vi "4-5 reverse.vi"() -> ()   [LabVIEW 2014]
doc: "This VI illustrates how to acquire a finite number of samples from a specified device. It requires the use of a microphone attached to the sound card. You can specify the number of samples to acquire, sample rate, number of channels and a bit rate per sample.\n------------------------------------\nAuther: Koji Ohashi\nCopyright (c) 2020 Japan LabVIEW Users Group, Volunteer members.\nThis VI is released under the MIT License.\nhttp://opensource.org/licenses/mit-license.php\n------------------------------------"
uses:
  <vilib>/sound2/lvsound2.llb/Sampling Mode.ctl
  <vilib>/sound2/lvsound2.llb/Sound Input Read (DBL).vi
  <vilib>/sound2/lvsound2.llb/Sound Output Write (DBL).vi
  <vilib>/sound2/lvsound2.llb/Sound Data Format.ctl
panel:
  out "Sound Output":waveform(dbl)[](graph)
  in  "Recording Time (sec)":dbl=5.0
  in  "Sound Format":T1={"sample rate (S/s)"=22050.0, "number of channels"=2, "bits per sample"=16}
  in  "device ID (Out)":u32
  in  "Device ID":u32
  out "Sound Input":waveform(dbl)[](graph)
  out "Number of Samples/ch":i32=10000
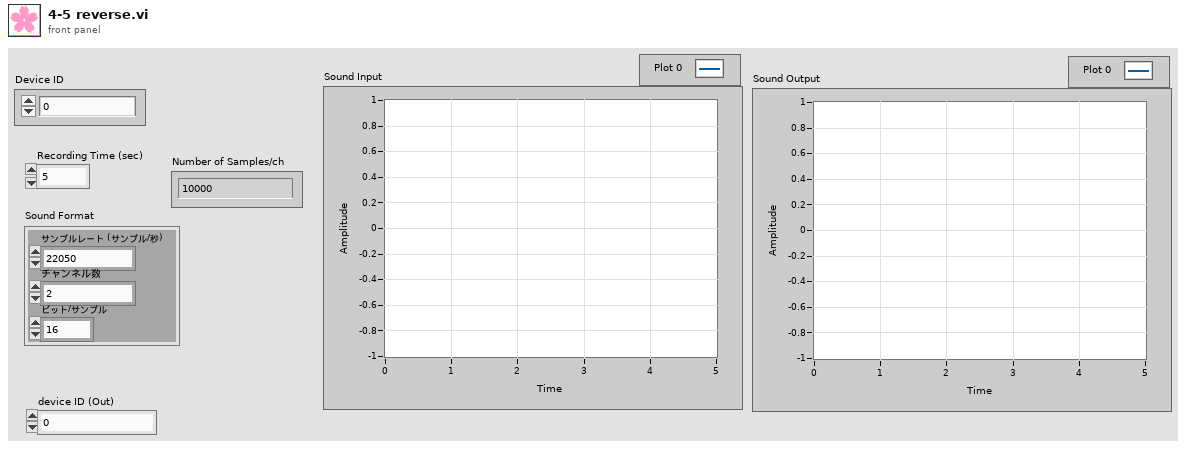
[diagram p1: front panel]
types:
  T1 = typedef "Sound Data Format.ctl" = cluster{"sample rate (S/s)":dbl, "number of channels":i32, "bits per sample":i32}
  T2 = typedef "Sampling Mode.ctl" = i32
  T3 = typedef "Sound Input Task ID.ctl" = u32
  T4 = typedef "Sound Output Task ID.ctl" = u32
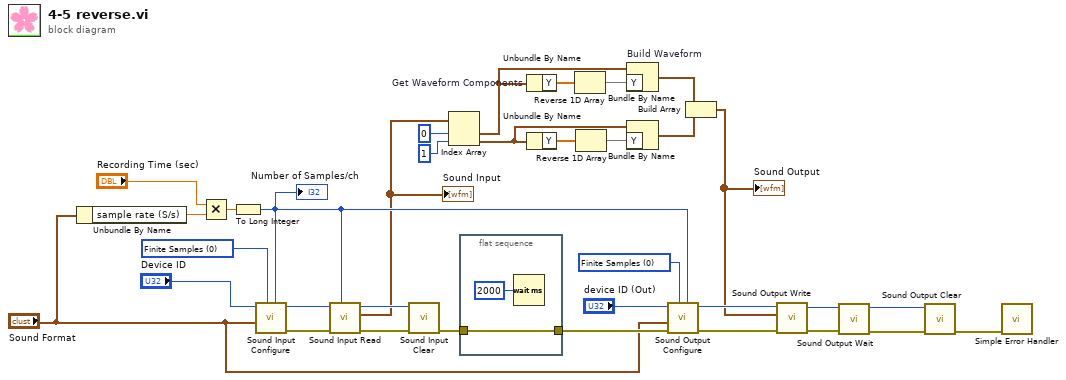
[diagram p0: block diagram]
diagram:
  w23 = T2 0 items=["Finite Samples", "Continuous Samples"] ("sample mode")
  w31 = T2 0 items=["Finite Samples", "Continuous Samples"] ("sample mode")
  n1 = Unbundle By Name("Sound Format") -> ("sample rate (S/s)"=w15:dbl)
  n2 = Multiply(x="Recording Time (sec)", y=w15) -> (x*y=w14:dbl)
  n3 = To Long Integer(number=w14) -> (32bit integer=w13:i32)
  "Number of Samples/ch" <- w13
  n4 = call <vilib>:"Sound Input Configure.vi"("number of samples/ch"=w13, "sample mode"=w31, "sound format"="Sound Format", "device ID"="Device ID") -> ("error out"=w34:errorcluster, "task ID"=w32:T3)  [unwired: 6 in]
  n5 = call-poly <vilib>:"Sound Input Read.vi"("number of samples/ch"=w13, "error in (no error)"=w34, "task ID"=w32) -> ("error out"=w29:errorcluster, "data"=w2:waveform(dbl)[], "task ID out"=w30:T3)  [unwired: 6 in]
  "Sound Input" <- w2
  n6 = call <vilib>:"Sound Input Clear.vi"("error in (no error)"=w29, "task ID"=w30) -> ("error out"=w28:errorcluster)  [unwired: 9 in]
  n7 = Index Array "Index Array"(array=w2, index #1=0 ("index"), index #2=1 ("index")) -> (element #1=w8:waveform(dbl), element #2=w6:waveform(dbl))
  n8 = flat-sequence {
    tunnel: w28 -> [w36]
    tunnel: [w36] -> w27
    frame #0 {
      n9 = Wait (ms)(milliseconds to wait=u32 2000) -> ()  [unwired: 1 out]
    }
  }
  n10 = Unbundle By Name "Get Waveform Components"(w8) -> ("Y"=w10:dbl[])
  n11 = Unbundle By Name(w6) -> ("Y"=w9:dbl[])
  n12 = Reverse 1D Array(array=w10) -> (reversed array=w7:dbl[])
  n13 = Reverse 1D Array(array=w9) -> (reversed array=w5:dbl[])
  n14 = Bundle By Name "Build Waveform"(cluster=w8, "Y"=w7) -> (w4:waveform(dbl))
  n15 = Bundle By Name(cluster=w6, "Y"=w5) -> (w3:waveform(dbl))
  n16 = call <vilib>:"Sound Output Configure.vi"("number of samples/ch"=w13, "sample mode"=w23, "error in (no error)"=w27, "sound format"="Sound Format", "device ID"="device ID (Out)") -> ("error out"=w24:errorcluster, "task ID"=w25:T4)  [unwired: 5 in]
  n17 = Build Array "Build Array"(w4, w3) -> (w1:waveform(dbl)[])
  "Sound Output" <- w1
  n18 = call-poly <vilib>:"Sound Output Write.vi"("error in (no error)"=w24, "data"=w1, "task ID"=w25) -> ("error out"=w22:errorcluster, "task ID out"=w21:T4)  [unwired: 7 in]
  n19 = call <vilib>:"Sound Output Wait.vi"("error in (no error)"=w22, "task ID"=w21) -> ("error out"=w19:errorcluster, "task ID out"=w20:T4)  [unwired: 8 in]
  n20 = call <vilib>:"Sound Output Clear.vi"("error in (no error)"=w19, "task ID"=w20) -> ("error out"=w18:errorcluster)  [unwired: 9 in]
  n21 = call <vilib>:"Simple Error Handler.vi"("error in (no error)"=w18) -> ()  [unwired: 4 in, 5 out]
